vi "lib String to Variant.vi"(8 "error in (no error)":errorcluster, 10 "String in":string, 11 "Variant":variant) -> (0 "error out":errorcluster, 3 "Variant out":variant)   [LabVIEW 2018]
uses:
  <vilib>/Utility/Data Type/Type Definitions/Data Type.ctl
  <vilib>/Utility/Data Type/NI_Data Type.lvlib
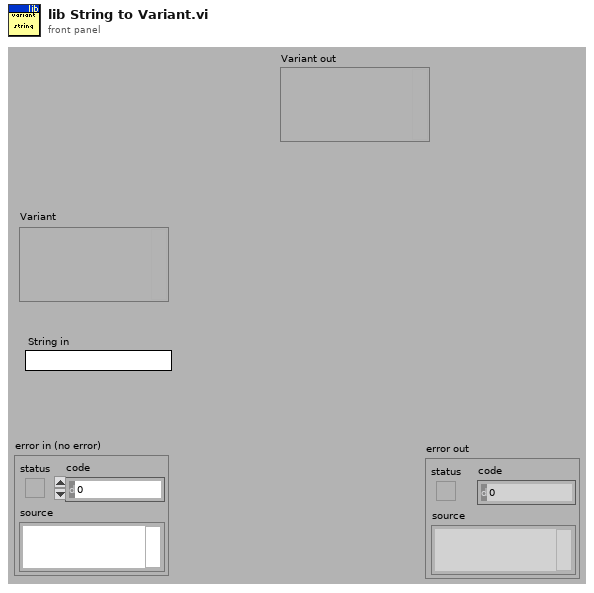
[diagram p1: front panel]
types:
  T1 = typedef "NI_Data Type.lvlib/Data Type.ctl" = enum8{"Invalid Type", "Void", "I8", "I16", "I32", "I64", "U8", "U16", "U32", "U64", "Single Float", "Double Float", "Extended Float", "Single Complex", "Double Complex", "Extended Complex", "Enum U8", "Enum U16", "Enum U32", "Enum U64", "Single Float With Unit", "Double Float With Unit", "Extended Float With Unit", "Single Complex with Unit", "Double Complex with Unit", "Extended Complex with Unit", "Boolean", "String", "Path", "Picture", "Tag", "Array", "Cluster", "Variant", "LV Variant", "Waveform", "Timestamp", "Digital Waveform", "Digital Data", "ExpressData", "Refnum", "External Data", "VI", "Poly VI", "LabVIEW Class Instance", "Fixed Point"}
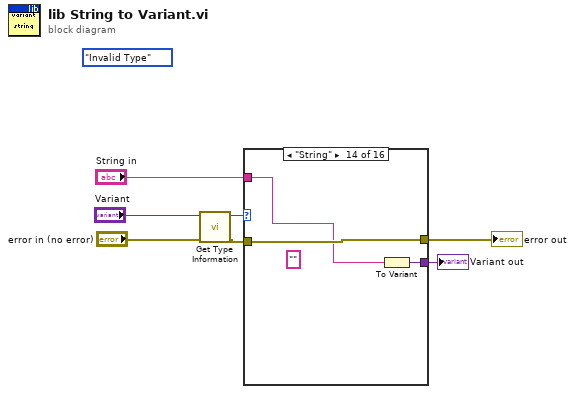
[diagram p0: block diagram]
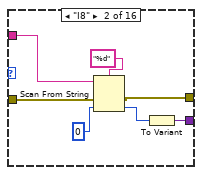
[diagram p3: hidden frame]
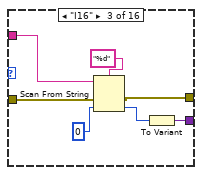
[diagram p4: hidden frame]
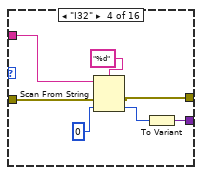
[diagram p5: hidden frame]
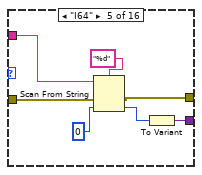
[diagram p6: hidden frame]
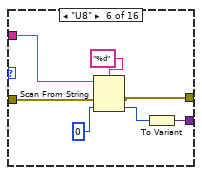
[diagram p7: hidden frame]
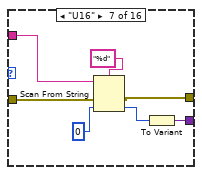
[diagram p8: hidden frame]
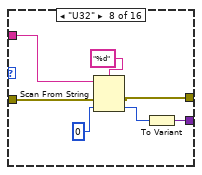
[diagram p9: hidden frame]
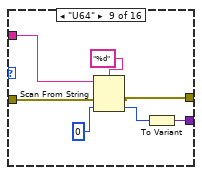
[diagram p10: hidden frame]
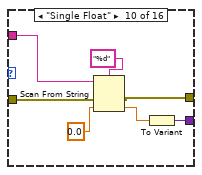
[diagram p11: hidden frame]
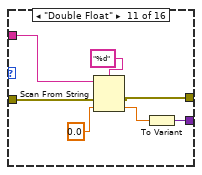
[diagram p12: hidden frame]
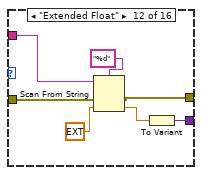
[diagram p13: hidden frame]
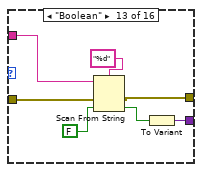
[diagram p14: hidden frame]
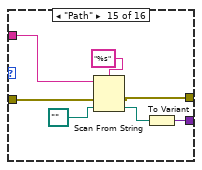
[diagram p15: hidden frame]
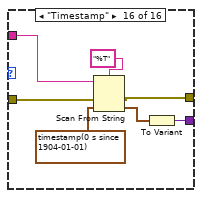
[diagram p16: hidden frame]
diagram:
  (unwired) Data_Type."Invalid Type" ("Type")
  n1 = call <vilib>:"Get Type Information.vi"("error in (no error)"="error in (no error)", "Variant"="Variant") -> ("error out"=w4:errorcluster, "Type"=w5:T1)  [unwired: 5 in, 3 out]
  n2 = case shown="\"String\"" w5 {
    tunnel: w4 -> [w8 w12 w19 w26 w33 w40 w47 w54 w61 w68 w75 w82 w90 w94 w100 w107]
    tunnel: [w8 w11 w18 w25 w32 w39 w46 w53 w60 w67 w74 w81 w89 w94 w99 w106] -> w3
    tunnel: [_ w10 w17 w24 w31 w38 w45 w52 w59 w66 w73 w80 w88 w95 w98 w105] -> w1
    tunnel: "String in" -> [_ w9 w16 w23 w30 w37 w44 w51 w58 w65 w72 w79 w87 w93 w97 w104]
    frame "Invalid Type", Default {
    }
    frame "I8" {
      n3 = Scan From String(format string="%d", input string=w9, error in=w12, default 1=i8 0) -> (error out=w11:errorcluster, output 1=w15:i8)  [unwired: 1 in, 2 out]
      n4 = To Variant(anything=w15) -> (Variant=w10:variant)
    }
    frame "I16" {
      n5 = Scan From String(format string="%d", input string=w16, error in=w19, default 1=i16 0) -> (error out=w18:errorcluster, output 1=w22:i16)  [unwired: 1 in, 2 out]
      n6 = To Variant(anything=w22) -> (Variant=w17:variant)
    }
    frame "I32" {
      n7 = Scan From String(format string="%d", input string=w23, error in=w26, default 1=0) -> (error out=w25:errorcluster, output 1=w29:i32)  [unwired: 1 in, 2 out]
      n8 = To Variant(anything=w29) -> (Variant=w24:variant)
    }
    frame "I64" {
      n9 = Scan From String(format string="%d", input string=w30, error in=w33, default 1=i64 0) -> (error out=w32:errorcluster, output 1=w36:i64)  [unwired: 1 in, 2 out]
      n10 = To Variant(anything=w36) -> (Variant=w31:variant)
    }
    frame "U8" {
      n11 = Scan From String(format string="%d", input string=w37, error in=w40, default 1=u8 0) -> (error out=w39:errorcluster, output 1=w43:u8)  [unwired: 1 in, 2 out]
      n12 = To Variant(anything=w43) -> (Variant=w38:variant)
    }
    frame "U16" {
      n13 = Scan From String(format string="%d", input string=w44, error in=w47, default 1=u16 0) -> (error out=w46:errorcluster, output 1=w50:u16)  [unwired: 1 in, 2 out]
      n14 = To Variant(anything=w50) -> (Variant=w45:variant)
    }
    frame "U32" {
      n15 = Scan From String(format string="%d", input string=w51, error in=w54, default 1=u32 0) -> (error out=w53:errorcluster, output 1=w57:u32)  [unwired: 1 in, 2 out]
      n16 = To Variant(anything=w57) -> (Variant=w52:variant)
    }
    frame "U64" {
      n17 = Scan From String(format string="%d", input string=w58, error in=w61, default 1=u64 0) -> (error out=w60:errorcluster, output 1=w64:u64)  [unwired: 1 in, 2 out]
      n18 = To Variant(anything=w64) -> (Variant=w59:variant)
    }
    frame "Single Float" {
      n19 = Scan From String(format string="%d", input string=w65, error in=w68, default 1=sgl 0.0) -> (error out=w67:errorcluster, output 1=w71:sgl)  [unwired: 1 in, 2 out]
      n20 = To Variant(anything=w71) -> (Variant=w66:variant)
    }
    frame "Double Float" {
      n21 = Scan From String(format string="%d", input string=w72, error in=w75, default 1=0.0) -> (error out=w74:errorcluster, output 1=w78:dbl)  [unwired: 1 in, 2 out]
      n22 = To Variant(anything=w78) -> (Variant=w73:variant)
    }
    frame "Extended Float" {
      n23 = Scan From String(format string="%d", input string=w79, error in=w82, default 1=ext 0.0) -> (error out=w81:errorcluster, output 1=w85:ext)  [unwired: 1 in, 2 out]
      n24 = To Variant(anything=w85) -> (Variant=w80:variant)
    }
    frame "Boolean" {
      n25 = Scan From String(format string="%d", input string=w87, error in=w90, default 1=FALSE) -> (error out=w89:errorcluster, output 1=w92:bool)  [unwired: 1 in, 2 out]
      n26 = To Variant(anything=w92) -> (Variant=w88:variant)
    }
    frame "String" {
      (unwired) ""
      n27 = To Variant(anything=w93) -> (Variant=w95:variant)
    }
    frame "Path" {
      n28 = Scan From String(format string="%s", input string=w97, error in=w100, default 1=path "") -> (error out=w99:errorcluster, output 1=w102:path)  [unwired: 1 in, 2 out]
      n29 = To Variant(anything=w102) -> (Variant=w98:variant)
    }
    frame "Timestamp" {
      n30 = Scan From String(format string="%T", input string=w104, error in=w107, default 1=timestamp(0 s since 1904-01-01)) -> (error out=w106:errorcluster, output 1=w109:timestamp)  [unwired: 1 in, 2 out]
      n31 = To Variant(anything=w109) -> (Variant=w105:variant)
    }
  }
  "error out" <- w3
  "Variant out" <- w1
